vi "Error Query.vi"(8 "error in (no error)":errorcluster, 11 "VISA resource name":refnum<visa-resource-name>) -> (0 "error out":errorcluster, 1 "Error Message":string, 2 "Error Code":i32[](array[numeric]), 3 "VISA resource name out":refnum<visa-resource-name>)   [LabVIEW 2012, in "ESP300.lvlib"]
doc: "Queries the instrument for any errors in the instrument's error queue. It will continue to read errors until all errors have been read from the instrument. Any errors will be returned in the <B>error out</B> control.\n\n<B>Note:</B>\nThis VI is called automatically by most driver VIs so it is not usually necessary to call this in an application."
uses:
  <instrlib>/ESP300/ESP300.lvlib
panel:
  # "EDIT: Note: The Error Query VI is included as a subVI in all driver VIs except low-level API VIs. If the instrument does not support error query, then remove the VI and remove subVI calls in each instrument driver VI that calls it."
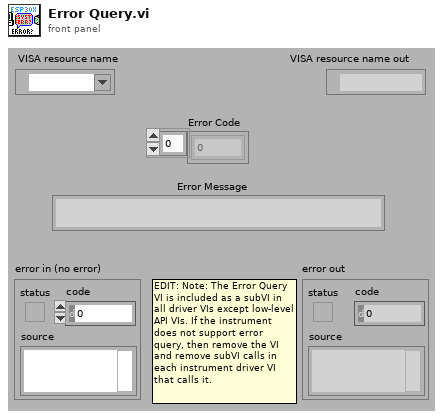
[diagram p1: front panel]
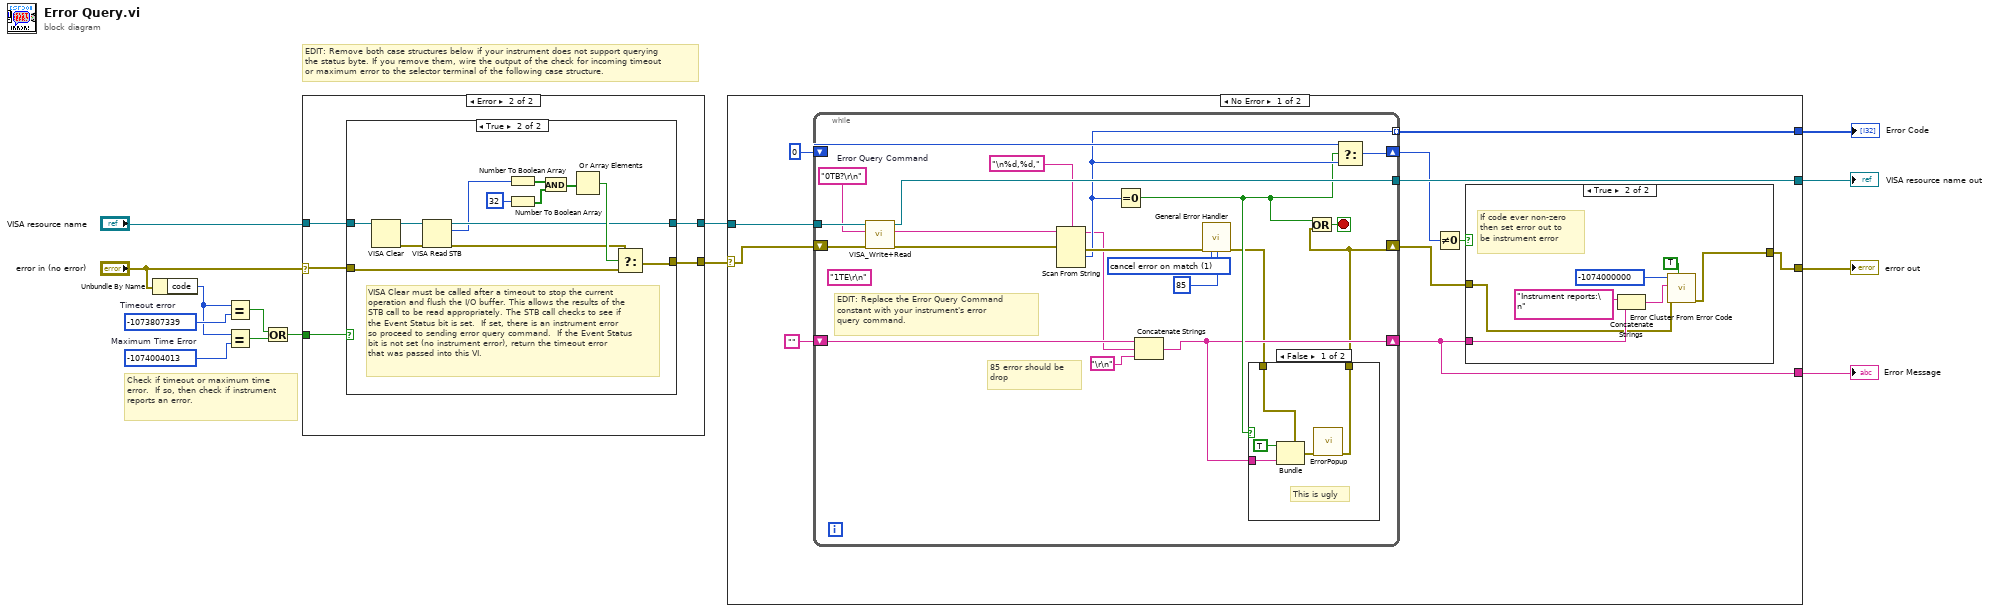
[diagram p0: block diagram]
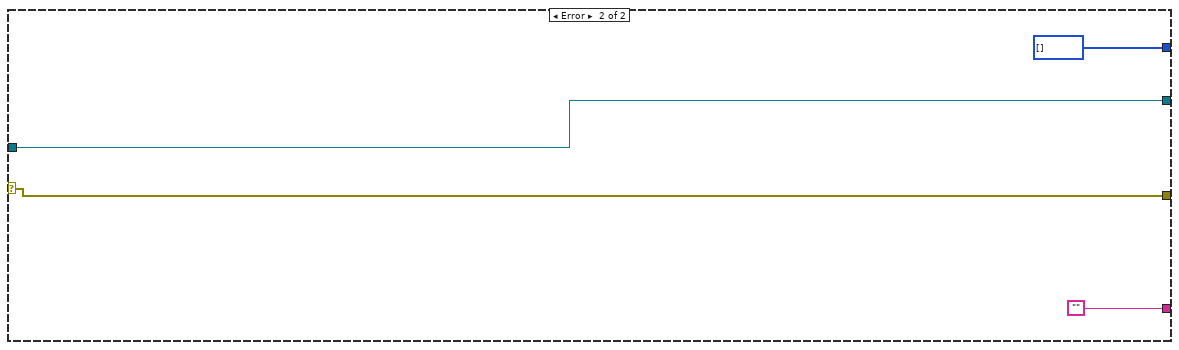
[diagram p6: hidden frame]
diagram:
  w5 = -1074004013  # Maximum Time Error
  w7 = -1073807339  # Timeout error
  # "Check if timeout or maximum time error.  If so, then check if instrument reports an error."
  # "EDIT: Remove both case structures below if your instrument does not support querying the status byte. If you remove them, wire the output of the check for incoming timeout or maximum error to the selector terminal of the following case structure."
  n1 = Unbundle By Name("error in (no error)") -> ("code"=w6:i32)
  n2 = Equal?(x=w6, y=w7) -> (x = y?=w3:bool)
  n3 = Equal?(x=w6, y=w5) -> (x = y?=w4:bool)
  n4 = Or(x=w3, y=w4) -> (x .or. y?=w2:bool)
  n5 = case shown="Error" "error in (no error)" {
    selector: "error in (no error)" -> [w15 w19]
    tunnel: "VISA resource name" -> [w16 w21]
    tunnel: [w16 w20] -> w9
    tunnel: [w15 w18] -> w10
    tunnel: w2 -> [_ w17]
    frame No Error {
    }
    frame Error {
      n6 = case shown="True" w17 {
        tunnel: w21 -> [w23 w29]
        tunnel: [w23 w26] -> w20
        tunnel: w19 -> [w22 w32]
        tunnel: [w22 w31] -> w18
        frame False {
          # "Error code not a timeout, so best to pass on to user."
        }
        frame True {
          # "VISA Clear must be called after a timeout to stop the current operation and flush the I/O buffer. This allows the results of the  STB call to be read appropriately. The STB call checks to see if the Event Status bit is set.  If set, there is an instrument error so proceed to sending error query command.  If the Event Status bit is not set (no instrument error), return the timeout error that was passed into this VI."
          n7 = VISA Clear(VISA resource name=w29) -> (VISA resource name out=w28:refnum<visa-resource-name>, error out=w27:errorcluster)  [unwired: 1 in]
          n8 = VISA Read STB(8:w27, 11:w28) -> (0:w25:errorcluster, 2:w24:u16, 3:w26:refnum<visa-resource-name>)
          n9 = Number To Boolean Array(number=w24) -> (Boolean array=w33:bool[])
          n10 = Number To Boolean Array(number=32) -> (Boolean array=w35:bool[])
          n11 = And(x=w33, y=w35) -> (x .and. y?=w34:bool[])
          n12 = Or Array Elements(Boolean array=w34) -> (logical OR=w30:bool)
          n13 = Select(t=w25, s=w30, f=w32) -> (s? t:f=w31:errorcluster)
        }
      }
    }
  }
  n14 = case shown="No Error" w10 {
    selector: w10 -> [w37 w83]
    tunnel: [w47 w86] -> w14
    tunnel: w9 -> [w46 w86]
    tunnel: [w42 w83] -> w13
    tunnel: [w40 ""] -> w12
    tunnel: [w39 i32[] []] -> w11
    frame No Error {
      n15 = while {
        tunnel: [w75] -> w47
        tunnel: w46 -> [w76]
        shift-right: [w60] -> w40
        shift-left: "" -> [w71]
        shift-right: [w68] -> w41
        shift-left: 0 -> [w69]
        shift-right: [w58] -> w38
        shift-left: w37 -> [w67]
        tunnel: [w63] -> w39 mode=indexing
        stop <- w72 stop-if-true
        (unwired) "1TE\r\n"
        w65 = 1 items=["no exception", "cancel error on match", "set error on match"] ("[exception action] (none:0)")
        w57 = "0TB?\r\n"  # Error Query Command
        # "85 error should be \ndrop"
        # "EDIT: Replace the Error Query Command\nconstant with your instrument's error\nquery command."
        n16 = call <instrlib>:"VISA_Write+Read.vi"("error in (no error)"=w67, "Write Buffer"=w57, "VISA resource name"=w76) -> ("error out"=w74:errorcluster, "readout"=w56:string, "VISA resource name out"=w75:refnum<visa-resource-name>)  [unwired: 6 in]
        n17 = Scan From String(format string="\n%d,%d,", input string=w56, error in=w74) -> (remaining string=w62:string, error out=w66:errorcluster, output 1=w63:i32)  [unwired: 4 in, 1 out]
        n18 = Equal To 0?(x=w63) -> (x = 0?=w61:bool)
        n19 = Concatenate Strings(w71, w62, "\r\n") -> (w60:string)
        n20 = call <vilib>:"General Error Handler.vi"("error in (no error)"=w66, "[exception action] (none:0)"=w65, "[exception code]"=85) -> ("error out"=w59:errorcluster)  [unwired: 8 in, 4 out]
        n21 = case shown="False" w61 {
          tunnel: w60 -> [w80 _]
          tunnel: w59 -> [w79 w82]
          tunnel: [w78 w82] -> w58
          frame False {
            # "This is ugly"
            n22 = Bundle(cluster=w79, "status"=TRUE, "source"=w80) -> (w81:errorcluster)  [unwired: 1 in]
            n23 = call <instrlib>:"ErrorPopup.vi"("error in (no error)"=w81) -> ("error out"=w78:errorcluster)  [unwired: 10 in]
          }
          frame True {
          }
        }
        n24 = Or(x=w61, y=w58) -> (x .or. y?=w72:bool)
        n25 = Select(t=w69, s=w61, f=w63) -> (s? t:f=w68:i32)
      }
      n26 = Not Equal To 0?(x=w41) -> (x != 0?=w43:bool)
      n27 = case shown="True" w43 {
        tunnel: w40 -> [_ w54]
        tunnel: [w48 w50] -> w42
        tunnel: w38 -> [w48 w49]
        frame False {
        }
        frame True {
          # "If code ever non-zero\nthen set error out to\nbe instrument error"
          n28 = Concatenate Strings("Instrument reports:\n" ("Source"), w54) -> (w51:string)
          n29 = call <vilib>:"Error Cluster From Error Code.vi"("show call chain? (False)"=TRUE, "error in (no error)"=w49, "error message (\"\")"=w51, "error code (0)"=-1074000000 ("Code")) -> ("error out"=w50:errorcluster)  [unwired: 5 in]
        }
      }
    }
    frame Error {
    }
  }
  "VISA resource name out" <- w14
  "error out" <- w13
  "Error Message" <- w12
  "Error Code" <- w11
